vi "ArmExecute.vi"   [LabVIEW 2020]
doc: "Execute Arm VI's\nInputs:\n\nOutputs:"
uses:
  <vilib>/Rock Robotics/WPI/Solenoid/WPI_SolenoidValue.ctl
  ArmGlobal.vi
  <vilib>/Rock Robotics/WPI/Solenoid/WPI_SolenoidSetEnum.vi
  <vilib>/Rock Robotics/WPI/ThirdParty/Phoenix-LabVIEW/Motor Controller/Controls/CTRE_Phoenix_MotorControl_ControlMode.ctl
types:
  T1 = typedef "WPI_SolenoidValue.ctl" = enum16{"Off", "On", "Forward", "Reverse"}
  T2 = typedef "WPI_SolenoidDevRef.ctl" = cluster{"DevStatus":errorcluster, "Pneumatics Control Module":u8, "Forward Solenoid Channel":T3, "Reverse Solenoid Channel":T3}
  T3 = typedef "WPI_SolenoidChannel.ctl" = enum8{"Solenoid 0", "Solenoid 1", "Solenoid 2", "Solenoid 3", "Solenoid 4", "Solenoid 5", "Solenoid 6", "Solenoid 7", "Solenoid 8", "Solenoid 9", "Solenoid 10", "Solenoid 11", "Solenoid 12", "Solenoid 13", "Solenoid 14", "Solenoid 15", "Invalid"}
  T4 = typedef "WPI_EncoderDevRef.ctl" = cluster{"DevStatus":errorcluster, "EncoderIndex":T5, "CounterIndex":T6, "DistancePerCount":dbl, "Decoding Type":T7}
  T5 = typedef "FPGA_EncoderIdx.ctl" = enum8{"Enc 0", "Enc 1", "Enc 2", "Enc 3", "Enc 4", "Enc 5", "Enc 6", "Enc 7", "Invalid"}
  T6 = typedef "FPGA_CounterCtrSystemIndex.ctl" = enum8{"Ctr 0", "Ctr 1", "Ctr 2", "Ctr 3", "Ctr 4", "Ctr 5", "Ctr 6", "Ctr 7", "Invalid"}
  T7 = typedef "WPI_EncoderType.ctl" = enum16{"1x", "2x", "4x"}
  T8 = typedef "WPI_MotorControlDeviceRef.ctl" = cluster{"DeviceStatus":errorcluster, "Type":T9, "PWM":cluster{"PWM Channel":T10, "DeadBand":T11}, "CAN":cluster{"Device Number":u8, "SetOutput VI Ref":variant, "GetOutput VI Ref":variant, "Enable VI Ref":variant, "Disable VI Ref":variant, "Data":variant}, "Invert":bool, "DIO PWM":cluster{"PWM \"Enable\" Channel":T10, "DIOChannel":T12, "PWM Rate":dbl}}
  T9 = typedef "WPI_MotorControlType.ctl" = enum16{"PWM", "CAN", "DIO PWM"}
  T10 = typedef "FPGA_DIOPWMChannel.ctl" = enum8{"PWM 0", "PWM 1", "PWM 2", "PWM 3", "PWM 4", "PWM 5", "PWM 6", "PWM 7", "PWM 8", "PWM 9", "PWM MXP 0", "PWM MXP 1", "PWM MXP 2", "PWM MXP 3", "PWM MXP 4", "PWM MXP 5", "PWM MXP 6", "PWM MXP 7", "PWM MXP 8", "PWM MXP 9", "Invalid"}
  T11 = typedef "WPI_PWMDeadband.ctl" = cluster{"Name":string, "maxPositivePwm":i32, "minPositivePwm":i32, "centerPwm":i32, "maxNegativePwm":i32, "minNegativePwm":i32, "angularRange":u16}
  T12 = typedef "FPGA_DIOChannel.ctl" = enum8{"DIO 0", "DIO 1", "DIO 2", "DIO 3", "DIO 4", "DIO 5", "DIO 6", "DIO 7", "DIO 8", "DIO 9", "DIO MXP 0", "DIO MXP 1", "DIO MXP 2", "DIO MXP 3", "DIO MXP 4", "DIO MXP 5", "DIO MXP 6", "DIO MXP 7", "DIO MXP 8", "DIO MXP 9", "DIO MXP 10", "DIO MXP 11", "DIO MXP 12", "DIO MXP 13", "DIO MXP 14", "DIO MXP 15", "SPI Port CS1", "SPI Port CS2", "SPI Port CS3", "SPI Port MISO", "SPI Port MOSI", "Invalid"}
  T13 = typedef "CTRE_Phoenix_MotorControl_ControlMode.ctl" = u16
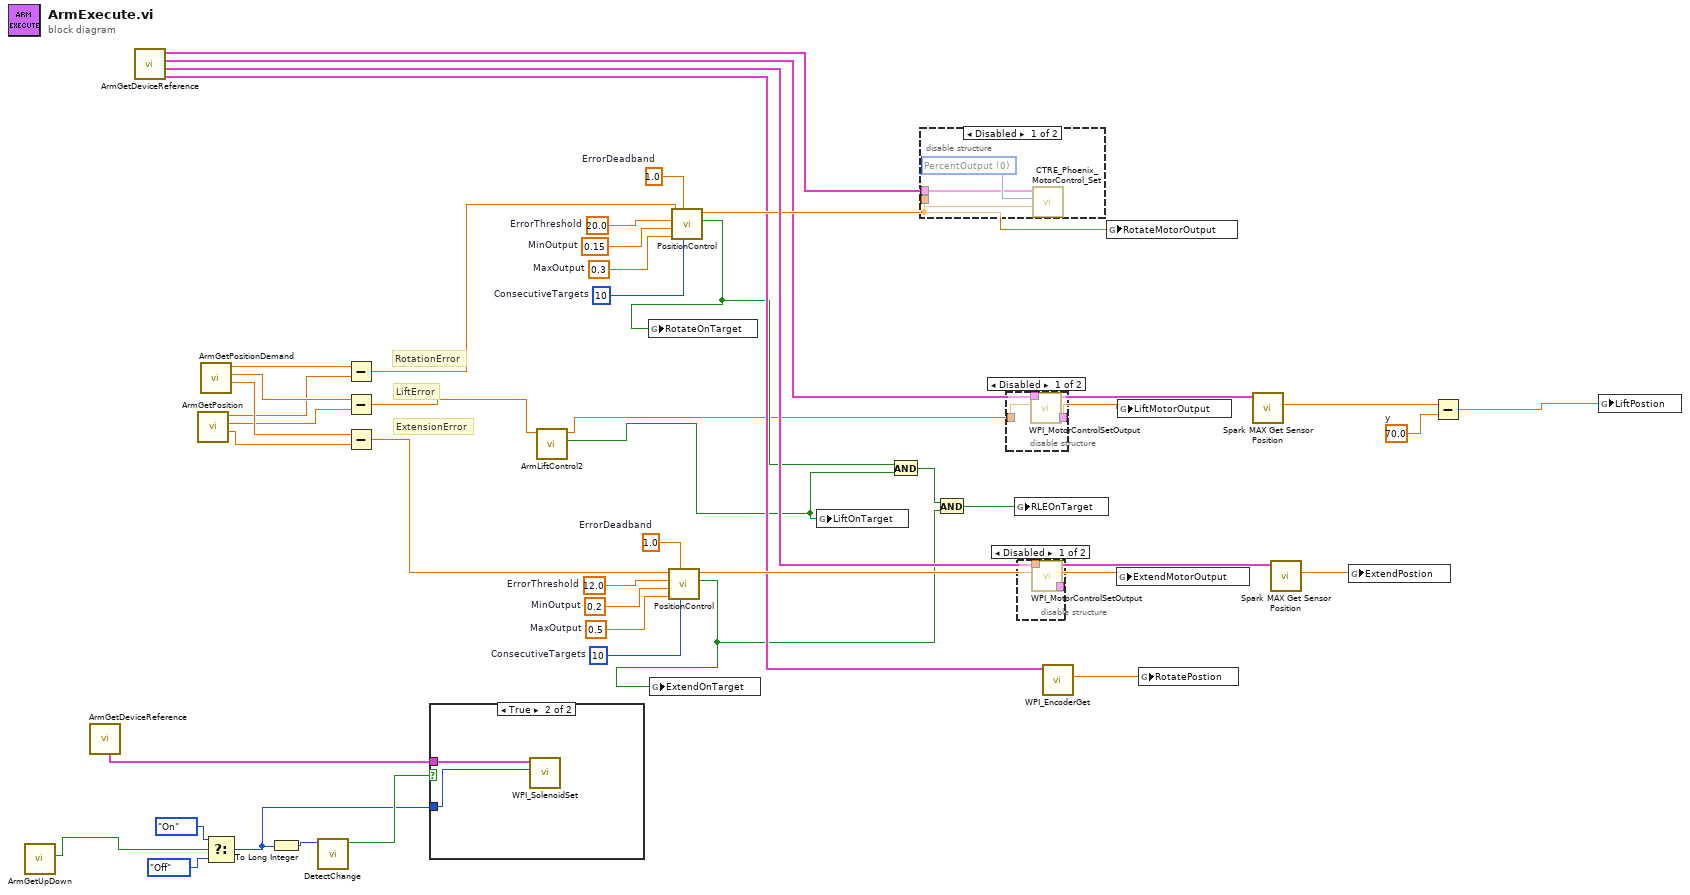
[diagram p0: block diagram]
diagram:
  w13 = 70.0  # y
  w28 = 10  # ConsecutiveTargets
  w29 = 0.5  # MaxOutput
  w30 = 0.2  # MinOutput
  w31 = 12.0  # ErrorThreshold
  w32 = 1.0  # ErrorDeadband
  w18 = 10  # ConsecutiveTargets
  w35 = 0.3  # MaxOutput
  w36 = 0.15  # MinOutput
  w37 = 20.0  # ErrorThreshold
  w38 = 1.0  # ErrorDeadband
  # "ExtensionError"
  # "LiftError"
  # "RotationError"
  n1 = call "ArmGetUpDown.vi"() -> ("ArmUpDown"=w1:bool)  [unwired: 11 in]
  n2 = call "ArmGetDeviceReference.vi"() -> ("ArmSolenoid"=w2:T2)  [unwired: 7 in, 4 out]
  n3 = call "ArmGetDeviceReference.vi"() -> ("armRotateEncoder"=w25:T4, "armExtend"=w41:T8, "armRotate"=w20:T8, "armLift"=w19:T8)  [unwired: 7 in, 1 out]
  n4 = call "ArmGetPosition.vi"() -> ("ExtendPostion"=w42:dbl, "LiftPostion"=w43:dbl, "RotatePostion"=w44:dbl)  [unwired: 9 in]
  n5 = call "ArmGetPositionDemand.vi"() -> ("ExtendPositonDemand(in)"=w45:dbl, "LiftPositionDemand(d)"=w46:dbl, "RotatePositonDemand(d)"=w47:dbl)  [unwired: 9 in]
  n6 = Select(t=WPI_SolenoidValue."On" ("Value"), s=w1, f=WPI_SolenoidValue."Off" ("Value")) -> (s? t:f=w4:T1)
  n7 = To Long Integer(number=w4) -> (32bit integer=w3:i32)
  n8 = call "DetectChange.vi"("Value"=w3) -> ("Changed"=w5:bool)  [unwired: 10 in]
  n9 = Subtract(x=w47, y=w44) -> (x-y=w33:dbl)
  n10 = Subtract(x=w46, y=w43) -> (x-y=w10:dbl)
  n11 = Subtract(x=w45, y=w42) -> (x-y=w27:dbl)
  n12 = case shown="True" w5 {
    tunnel: w2 -> [_ w49]
    tunnel: w4 -> [_ w48]
    frame False {
    }
    frame True {
      n13 = call-poly <vilib>:"WPI_SolenoidSet.vi"("Value"=w48, "SolenoidDevRef"=w49) -> ()  [unwired: 8 in, 2 out]
    }
  }
  n14 = call "ArmLiftControl2.vi"("erronIn(d)"=w10) -> ("OnTarget"=w8:bool, "motorOutput"=w9:dbl)  [unwired: 9 in]
  n15 = call "PositionControl.vi"("ConsecutiveTargets"=w28, "ErrorDeadband"=w32, "MaxOutput"=w29, "MinOutput"=w30, "ErrorThreshold"=w31, "Error"=w27) -> ("OnTarget"=w16:bool, "OutputValue"=w26:dbl)  [unwired: 3 in, 1 out]
  n16 = global write "ArmGlobal.vi" "ExtendOnTarget"(w16) -> ()
  n17 = call "PositionControl.vi"("ConsecutiveTargets"=w18, "ErrorDeadband"=w38, "MaxOutput"=w35, "MinOutput"=w36, "ErrorThreshold"=w37, "Error"=w33) -> ("OnTarget"=w15:bool, "OutputValue"=w34:dbl)  [unwired: 3 in, 1 out]
  n18 = global write "ArmGlobal.vi" "RotateOnTarget"(w15) -> ()
  n19 = global write "ArmGlobal.vi" "LiftOnTarget"(w8) -> ()
  n20 = And(x=w15, y=w8) -> (x .and. y?=w17:bool)
  n21 = disable-structure shown="Disabled" {
    disable-tunnel: w34 -> [w52 _]
    disable-tunnel: w19 -> [w50 _]
    frame Disabled {
      w51 = T13 0 items=["PercentOutput"=0, "Position"=1, "Velocity"=2, "Current"=3, "Follower"=5, "MotionProfile"=6, "MotionMagic"=7, "MotionProfileArc"=10, "Disabled"=15] ("Control Mode")
      n22 = call <vilib>:"CTRE_Phoenix_MotorControl_Set.vi"("Output"=w52, "Control Mode"=w51, "PhoenixMotorControlDevRef"=w50) -> ()  [unwired: 7 in, 2 out]
    }
    frame Enabled {
    }
  }
  n23 = And(x=w17, y=w16) -> (x .and. y?=w14:bool)
  n24 = disable-structure shown="Disabled" {
    disable-tunnel: w9 -> [w56 _]
    disable-tunnel: [w55 _] -> w39
    disable-tunnel: [w54 _] -> w22
    disable-tunnel: w20 -> [w53 _]
    frame Disabled {
      n25 = call <vilib>:"WPI_MotorControlSetOutput.vi"("Output"=w56, "MotorControlDevRef"=w53) -> ("Motor Output"=w55:dbl, "MotorControlDevRef"=w54:T8)  [unwired: 7 in, 1 out]
    }
    frame Enabled {
    }
  }
  n26 = global write "ArmGlobal.vi" "RLEOnTarget"(w14) -> ()
  n27 = disable-structure shown="Disabled" {
    disable-tunnel: w41 -> [w60 _]
    disable-tunnel: [w59 _] -> w40
    disable-tunnel: w26 -> [w58 _]
    disable-tunnel: [w57 _] -> w23
    frame Disabled {
      n28 = call <vilib>:"WPI_MotorControlSetOutput.vi"("Output"=w58, "MotorControlDevRef"=w60) -> ("Motor Output"=w59:dbl, "MotorControlDevRef"=w57:T8)  [unwired: 7 in, 1 out]
    }
    frame Enabled {
    }
  }
  n29 = call <vilib>:"WPI_EncoderGet.vi"("EncoderDevRef"=w25) -> ("Distance"=w24:dbl)  [unwired: 5 in, 5 out]
  n30 = global write "ArmGlobal.vi" "RotateMotorOutput"(w34) -> ()
  n31 = global write "ArmGlobal.vi" "ExtendMotorOutput"(w40) -> ()
  n32 = global write "ArmGlobal.vi" "LiftMotorOutput"(w39) -> ()
  n33 = global write "ArmGlobal.vi" "RotatePostion"(w24) -> ()
  n34 = call <vilib>:"Spark MAX Get Sensor Position.vi"("MotorControlDevRef in"=w22) -> ("Sensor Position"=w12:dbl)  [unwired: 7 in, 3 out]
  n35 = call <vilib>:"Spark MAX Get Sensor Position.vi"("MotorControlDevRef in"=w23) -> ("Sensor Position"=w21:dbl)  [unwired: 7 in, 3 out]
  n36 = global write "ArmGlobal.vi" "ExtendPostion"(w21) -> ()
  n37 = Subtract(x=w12, y=w13) -> (x-y=w11:dbl)
  n38 = global write "ArmGlobal.vi" "LiftPostion"(w11) -> ()
